vi "SVPO Convert to Even Angle Signal (N Ch DBL WDT).vi"(0 "scaled signals [EU]":waveform(dbl)[](array[waveform]), 2 "reset? (F)":bool, 7 "speed position info":T1, 12 "max order":dbl=16.0) -> (4 "even-angle signals":cluster{"r0":dbl, "dr":dbl, "Y":dbl[]}[](array[cluster]) {"r0" format="%.2p"; "dr" format="%.2p"; "Y" format="%.2f"}, 8 "even-angle position info":T1)   [LabVIEW 2017, in "SoundVib_OrderTracking.lvlib"]
doc: "Converts an even-time-spaced scaled signal to an even-angle-spaced signal by resampling the acquired signal. The output signal is synchronous to the rotational speed with a constant number of samples per revolution. Use this VI on embedded targets that have limited computational resources. Wire data to the <B>scaled signal [EU]</B> input to determine the polymorphic instance to use or manually select the instance."
uses:
  <vilib>/addons/Sound and Vibration/Order Analysis/Resample Order Tracking/SoundVib_OrderTracking.lvlib
  <vilib>/addons/Sound and Vibration/Order Analysis/Misc/OAT Position Info.ctl
  <vilib>/addons/Sound and Vibration/Order Analysis/Adv Resampling/sv_Prepare Resample Data (DBL Array).vi
  <vilib>/addons/Sound and Vibration/Order Analysis/Adv Resampling/sv_Build Even Angle Signal (N Channels).vi
  <vilib>/addons/Sound and Vibration/Order Analysis/Resample Order Tracking/SubVIs/sv_Convert to Even Angle Signal (Generic) with IC.vi
  <vilib>/addons/Sound and Vibration/Order Analysis/Adv Resampling/oa_CIC Interpolation Filter with IC.vi
  <vilib>/addons/Sound and Vibration/Order Analysis/Adv Resampling/sv_Resample (Const to Variable, DBL Array) with IC.vi
  <vilib>/addons/Sound and Vibration/Order Analysis/Adv Resampling/sv_Resample Filter Prototype Design.vi
  <vilib>/addons/Sound and Vibration/Order Analysis/Adv Resampling/oa_Adjust Resample State Info.vi
  <vilib>/addons/Sound and Vibration/Order Analysis/Adv Resampling/OAT LP Kaiser Window Design.vi
  <vilib>/addons/Sound and Vibration/Order Analysis/Resample Order Tracking/SubVIs/oa_CIC Filter Length.vi
  <vilib>/addons/Sound and Vibration/Order Analysis/Adv Resampling/sv_Get Actual Max Order.vi
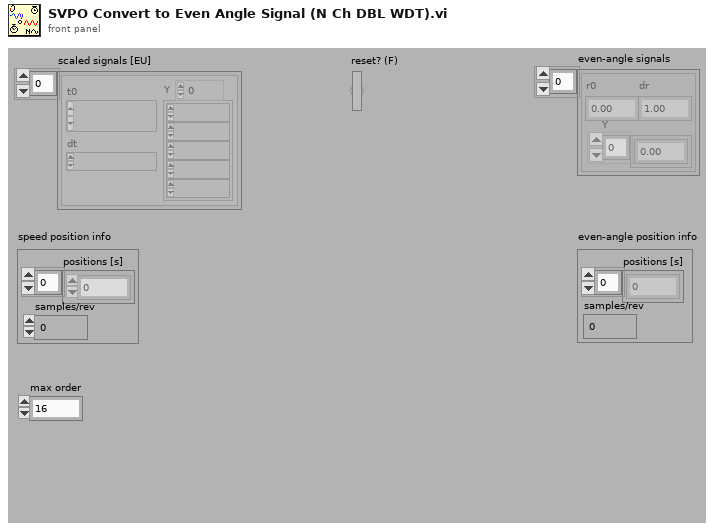
[diagram p1: front panel]
types:
  T1 = typedef "OAT Position Info.ctl" = cluster{"positions [s]":dbl[], "samples/rev":dbl}
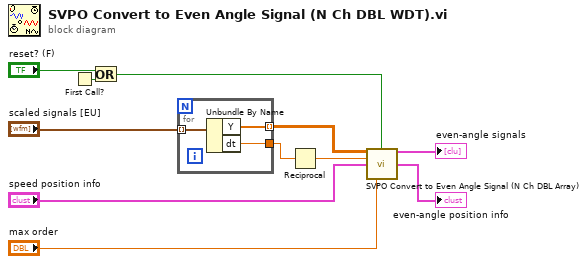
[diagram p0: block diagram]
diagram:
  n1 = First Call?() -> (First Call?: T/F=w10:bool)
  n2 = Or(x="reset? (F)", y=w10) -> (x .or. y?=w5:bool)
  n3 = for {
    tunnel: "scaled signals [EU]" -> [w14] mode=indexing
    tunnel: [w13] -> w6 mode=indexing
    tunnel: [w12] -> w8
    n4 = Unbundle By Name(w14) -> ("Y"=w13:dbl[], "dt"=w12:dbl)
  }
  n5 = Reciprocal(x=w8) -> (1/x=w7:dbl)
  n6 = call <vilib>:"SVPO Convert to Even Angle Signal (N Ch DBL Array).vi"("scaled signals [EU]"=w6, "reset? (F)"=w5, "sampling rate [Hz]"=w7, "speed position info"="speed position info", "max order"="max order") -> ("even-angle signals"=→"even-angle signals":cluster{"r0":dbl, "dr":dbl, "Y":dbl[]}[], "even-angle position info"=→"even-angle position info":T1)  [unwired: 9 in]
